vi "flow-IRR.vi"(10 "_UV Sample Interval Seconds":u16, 11 "Irrigation Dose Time":u16) -> (2 "_UV Flow":T1[](array[typedef]), 3 "IRR Flow":T1[](array[typedef]))   [LabVIEW 2024]
uses:
  controls/UiStepBuilder.ctl
  controls/type.step-builder.ctl
panel:
  # "e"
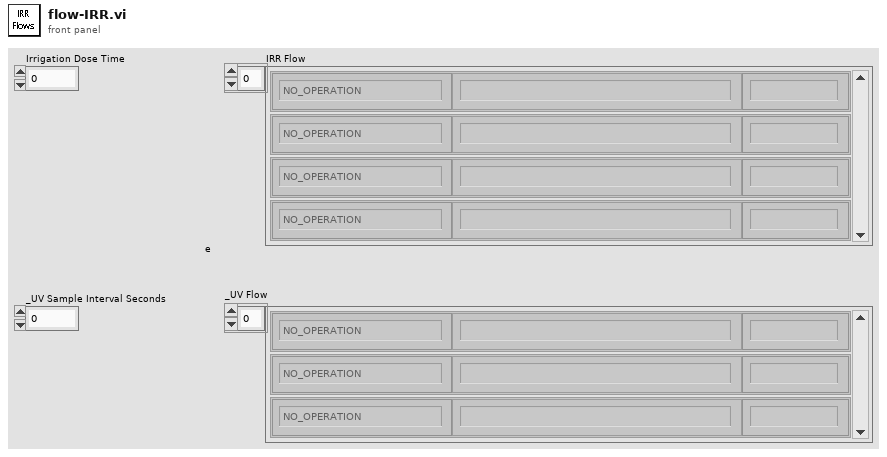
[diagram p1: front panel]
types:
  T1 = typedef "UiStepBuilder.ctl" = cluster{"Step Function":T2, "ParamString":string, "Step Label":string}
  T2 = typedef "type.step-builder.ctl" = enum16{"NO_OPERATION", "DELAY-JUMP", "DELAY", "JUMP", "COMPLETE", "SCHEDULER", "IRR-CHECK", "UNIT-CHECK", "UNIT-SAMPLE", "UNIT-DOSE", "LOG-REPORT", "LOG-MESSAGE", "IO-READ", "IO-READ-MANY", "IO-WRITE", "IO-COMPARE-OUT", "IO-COMPARE-IN", "PROC-START", "PROC-STOP", "PROC-LOAD", "PROC-IS-COMPLETED", "RECORD-MOVE", "GET-RH", "GET-UV", "GET-WD", "GET-WS", "OCS-CHECK", "OCS-RECORD"}
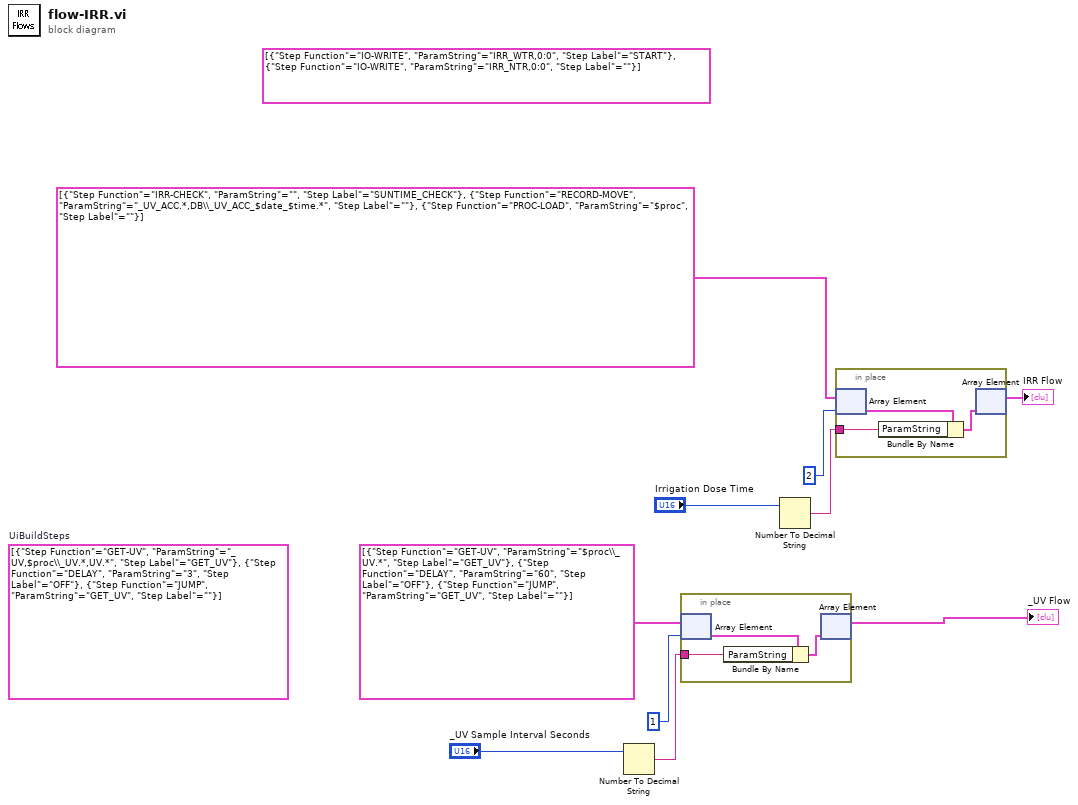
[diagram p0: block diagram]
diagram:
  (unwired) T1[] [{"Step Function"=enum."IO-WRITE", "ParamString"="IRR_WTR,0:0", "Step Label"="START"}, {"Step Function"=enum."IO-WRITE", "ParamString"="IRR_NTR,0:0", "Step Label"=""}] ("Irrigation Flow")
  (unwired) T1[] [{"Step Function"=enum."GET-UV", "ParamString"="_UV,$proc\\_UV.*,UV.*", "Step Label"="GET_UV"}, {"Step Function"=enum."DELAY", "ParamString"="3", "Step Label"="OFF"}, {"Step Function"=enum."JUMP", "ParamString"="GET_UV", "Step Label"=""}]  # UiBuildSteps
  n1 = Number To Decimal String(number="_UV Sample Interval Seconds") -> (decimal integer string=w3:string)  [unwired: 1 in]
  n2 = in-place {
    in-place-border: w3 -> [w12]
    n3 = in-place-array #1(T1[] [{"Step Function"=enum."GET-UV", "ParamString"="$proc\\_UV.*", "Step Label"="GET_UV"}, {"Step Function"=enum."DELAY", "ParamString"="60", "Step Label"="OFF"}, {"Step Function"=enum."JUMP", "ParamString"="GET_UV", "Step Label"=""}] ("UiBuildSteps"), 1) -> (w13:T1)
    n4 = Bundle By Name(cluster=w13, "ParamString"=w12) -> (w11:T1)
    n5 = in-place-array #1(w11) -> (→"_UV Flow":T1[])  [unwired: 1 out]
  }
  n6 = Number To Decimal String(number="Irrigation Dose Time") -> (decimal integer string=w7:string)  [unwired: 1 in]
  n7 = in-place {
    in-place-border: w7 -> [w15]
    n8 = in-place-array #2(T1[] [{"Step Function"=enum."IRR-CHECK", "ParamString"="", "Step Label"="SUNTIME_CHECK"}, {"Step Function"=enum."RECORD-MOVE", "ParamString"="_UV_ACC.*,DB\\_UV_ACC_$date_$time.*", "Step Label"=""}, {"Step Function"=enum."PROC-LOAD", "ParamString"="$proc", "Step Label"=""}] ("Irrigation Flow"), 2) -> (w16:T1)
    n9 = Bundle By Name(cluster=w16, "ParamString"=w15) -> (w14:T1)
    n10 = in-place-array #2(w14) -> (→"IRR Flow":T1[])  [unwired: 1 out]
  }
